vi "calc timeout.vi"(10 "init options":T12={"UI visible?"=FALSE, "Update rate (ms)"=250, "Sidebar.Visible"=TRUE, "time to plot (init)"=600.0, "time to plot (max)"=inf, "config file start path"=path "", "Title.Visible"=TRUE, "Title"="Title", "TimeZone"=enum."Local"} {"time to plot (init)" format="%<%H:%M:%S>t"}, 11 "Loop data in":T1={"TitleCollapse"=refnum, "MouseDownState"=enum."Idle", "RightClickCache"={"Mod"={"Ctrl"=FALSE, "Shift"=FALSE}, "CoordsStart"={"Horizontal"=0, "Vertical"=0}, "CoordsEnd"={"Horizontal"=0, "Vertical"=0}, "PlotAreaBounds"={"Left"=10, "Top"=10, "Right"=0, "Bottom"=0}, "slice"=[]}, "ZoomCache"={"SuppressedPlots"=[], "LeftAxis"={"NeedsRevert?"=FALSE, "Scale Fit"=0, "Range"={"Minimum"=0.0, "Maximum"=0.0, "Increment"=0.0, "Minor Increment"=0.0, "Start"=0.0}}, "RightAxis"={"NeedsRevert?"=FALSE, "Scale Fit"=0, "Range"={"Minimum"=0.0, "Maximum"=0.0, "Increment"=0.0, "Minor Increment"=0.0, "Start"=0.0}}, "Mod"={"Shift"=FALSE}}, "UpdateTime"=0.0, "keyboard"=refnum, "visible?"=FALSE}) -> (2 "Update?":bool, 3 "timeout":i32)   [LabVIEW 2021, in "RocketPlot.lvlib"]
uses:
  RocketPlot.lvlib
  Classes/RocketPlotHandle/SubVIs/Init Options.ctl
  TypeDefs/TimeZone.ctl
  TypeDefs/plot while loop data.ctl
  CollapsePanel/CollapsePanel.lvclass
  TypeDefs/MouseDownState.ctl
  TypeDefs/RightClickCache.ctl
  TypeDefs/RightClickCache PlatMod.ctl
  <vilib>/Utility/miscctls.llb/LVPoint32TypeDef.ctl
  <vilib>/Utility/miscctls.llb/LVRectTypeDef.ctl
  TypeDefs/Slice average.ctl
  TypeDefs/ZoomCache.ctl
  TypeDefs/RangeCache.ctl
  <vilib>/Utility/miscctls.llb/LVRangeTypeDef.ctl
  TypeDefs/ZoomCache PlatMod.ctl
  Classes/RocketPlotHandle/RocketPlotHandle.lvclass
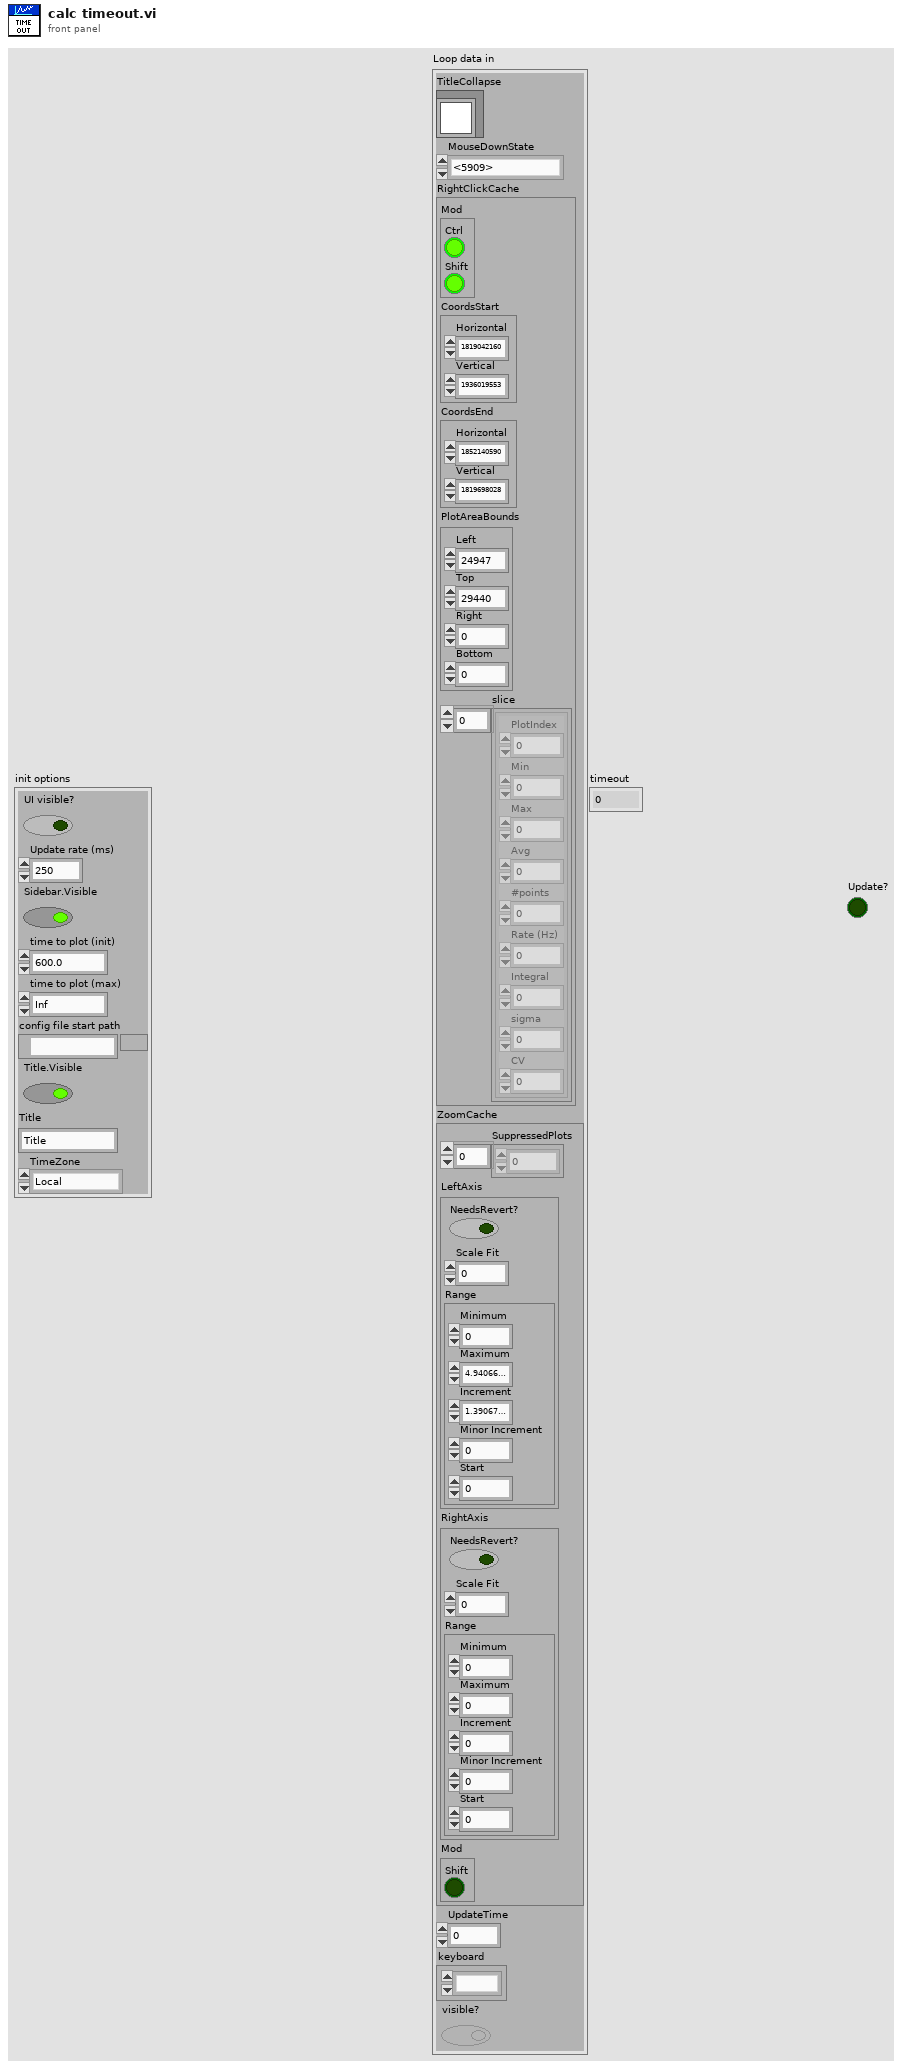
[diagram p1: front panel]
types:
  T1 = typedef "RocketPlot.lvlib/plot while loop data.ctl" = cluster{"TitleCollapse":refnum<class "CollapsePanel.lvclass">, "MouseDownState":T2, "RightClickCache":T3, "ZoomCache":T8, "UpdateTime":dbl, "keyboard":refnum<k1>, "visible?":bool}
  T2 = typedef "RocketPlot.lvlib/MouseDownState.ctl" = enum16{"Idle", "Pan", "Zoom", "Zoom-Post", "RightClick"}
  T3 = typedef "RocketPlot.lvlib/RightClickCache.ctl" = cluster{"Mod":T4, "CoordsStart":T5, "CoordsEnd":T5, "PlotAreaBounds":T6, "slice":T7[]}
  T4 = typedef "RocketPlot.lvlib/RightClickCache PlatMod.ctl" = cluster{"Ctrl":bool, "Shift":bool}
  T5 = typedef "LVPoint32TypeDef.ctl" = cluster{"Horizontal":i32, "Vertical":i32}
  T6 = typedef "LVRectTypeDef.ctl" = cluster{"Left":i16, "Top":i16, "Right":i16, "Bottom":i16}
  T7 = typedef "RocketPlot.lvlib/Slice average.ctl" = cluster{"PlotIndex":i32, "Min":dbl, "Max":dbl, "Avg":dbl, "#points":u32, "Rate (Hz)":dbl, "Integral":dbl, "sigma":dbl, "CV":dbl}
  T8 = typedef "RocketPlot.lvlib/ZoomCache.ctl" = cluster{"SuppressedPlots":i32[], "LeftAxis":T9, "RightAxis":T9, "Mod":T11}
  T9 = typedef "RocketPlot.lvlib/RangeCache.ctl" = cluster{"NeedsRevert?":bool, "Scale Fit":u8, "Range":T10}
  T10 = typedef "LVRangeTypeDef.ctl" = cluster{"Minimum":dbl, "Maximum":dbl, "Increment":dbl, "Minor Increment":dbl, "Start":dbl}
  T11 = typedef "RocketPlot.lvlib/ZoomCache PlatMod.ctl" = cluster{"Shift":bool}
  T12 = typedef "RocketPlotHandle.lvclass/Init Options.ctl" = cluster{"UI visible?":bool, "Update rate (ms)":u32, "Sidebar.Visible":bool, "time to plot (init)":dbl, "time to plot (max)":dbl, "config file start path":path, "Title.Visible":bool, "Title":string, "TimeZone":T13}
  T13 = typedef "RocketPlot.lvlib/TimeZone.ctl" = enum16{"UTC", "Local"}
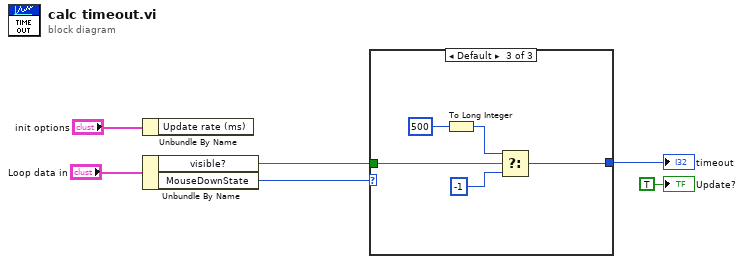
[diagram p0: block diagram]
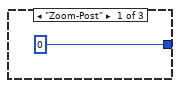
[diagram p2: hidden frame]
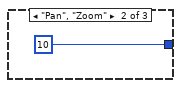
[diagram p3: hidden frame]
diagram:
  n1 = Unbundle By Name("init options") -> ()  [unwired: 1 out]
  n2 = Unbundle By Name("Loop data in") -> ("visible?"=w4:bool, "MouseDownState"=w2:T2)
  n3 = case shown="Default" w2 {
    tunnel: w4 -> [_ _ w11]
    tunnel: [0 ("32bit integer") 10 ("32bit integer") w10] -> w3
    frame "Zoom-Post" {
    }
    frame "Pan", "Zoom" {
    }
    frame Default {
      n4 = To Long Integer(number=500) -> (32bit integer=w13:i32)
      n5 = Select(t=w13, s=w11, f=-1 ("32bit integer")) -> (s? t:f=w10:i32)
    }
  }
  "timeout" <- w3
  "Update?" <- TRUE ("Update?")
